vi "GenTest.vi"() -> ()   [LabVIEW 2017]
uses:
  DG822.lvlib
panel:
  out "Result":string
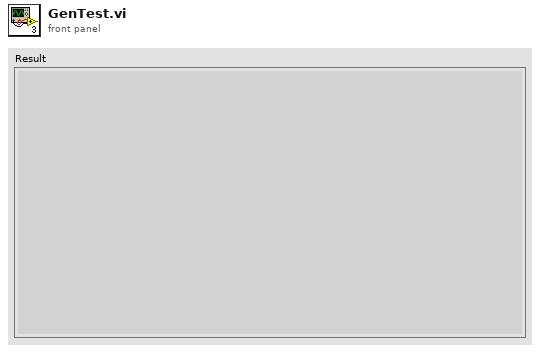
[diagram p1: front panel]
types:
  T1 = enum16{"SIN", "SQU", "RAMP", "PULSE", "NOISE", "HARM"}
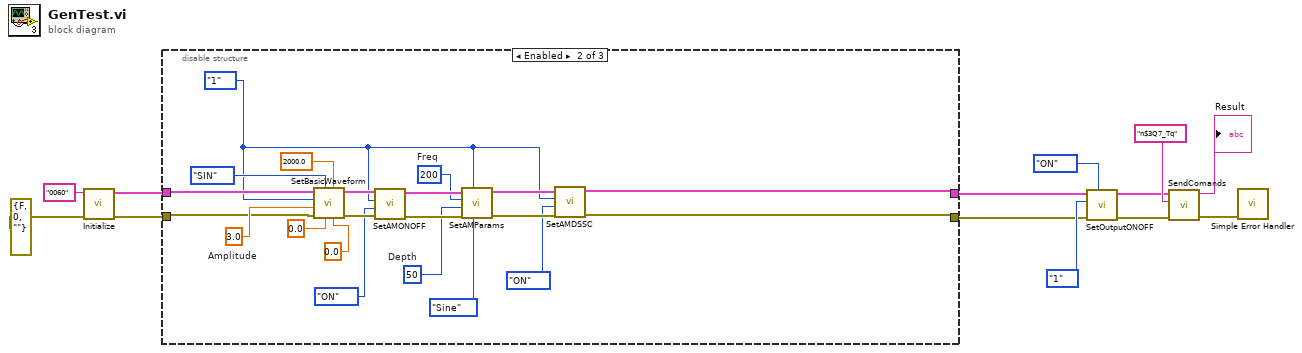
[diagram p0: block diagram]
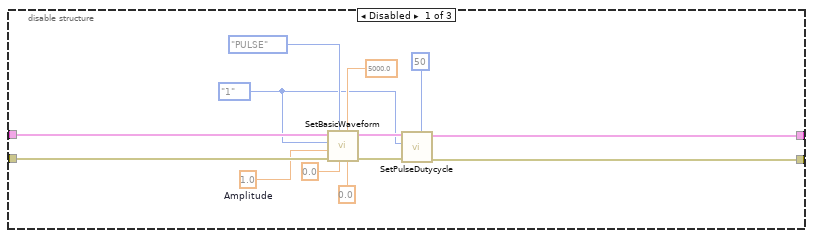
[diagram p2: hidden frame]
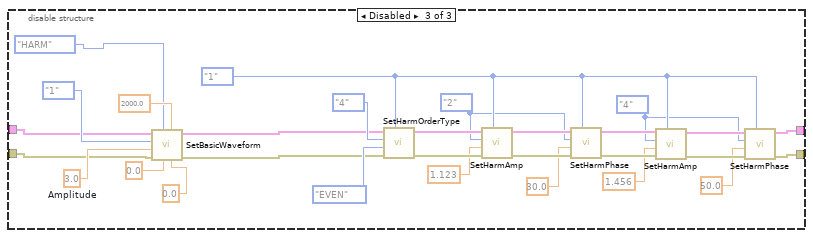
[diagram p3: hidden frame]
diagram:
  n1 = call "Initialize.vi"("error in (no error)"=errorcluster {"status"=FALSE, "code"=0, "source"=""}, "UserID"="0060") -> ("error out"=w7:errorcluster, "OutData"=w8:cluster{string, "userdata":string})  [unwired: 8 in]
  n2 = disable-structure shown="Enabled" {
    disable-tunnel: w8 -> [w26 w42 w53]
    disable-tunnel: w7 -> [w25 w41 w52]
    disable-tunnel: [w18 w34 w66] -> w2
    disable-tunnel: [w16 w33 w65] -> w1
    frame Disabled {
      w22 = 1.0  # Amplitude
      w15 = enum16{"1", "2"}."1" ("Source")
      n3 = call "SetBasicWaveform.vi"("Phase"=0.0, "Frequency"=5000.0, "Offset"=0.0, "Waveform"=enum16{"SIN", "SQU", "RAMP", "PULSE", "NOISE"}."PULSE", "error in"=w25, "Amplitude"=w22, "Source"=w15, "InputData"=w26) -> ("error out"=w17:errorcluster, "OutputData"=w19:cluster{"String":string, string})  [unwired: 2 in]
      n4 = call "SetPulseDutycycle.vi"("Dutycycle"=u8 50, "error in"=w17, "Source"=w15, "InputData"=w19) -> ("error out"=w16:errorcluster, "OutputData"=w18:cluster{"String":string, string})  [unwired: 6 in]
    }
    frame Enabled {
      w28 = u8 50  # Depth
      w30 = u32 200  # Freq
      w43 = 3.0  # Amplitude
      w32 = enum16{"1", "2"}."1" ("Source")
      n5 = call "SetBasicWaveform.vi"("Phase"=0.0, "Frequency"=2000.0, "Offset"=0.0, "Waveform"=T1."SIN", "error in"=w41, "Amplitude"=w43, "Source"=w32, "InputData"=w42) -> ("error out"=w39:errorcluster, "OutputData"=w40:cluster{"String":string, string})  [unwired: 2 in]
      n6 = call "SetAMONOFF.vi"("error in"=w39, "State"=enum16{"OFF", "ON"}."ON", "Source"=w32, "InputData"=w40) -> ("error out"=w37:errorcluster, "OutputData"=w38:cluster{"String":string, string})  [unwired: 6 in]
      n7 = call "SetAMParams.vi"("Func"=enum16{"Sine", "Square", "Trianle"}."Sine", "Source"=w32, "error in"=w37, "Depth"=w28, "Freq"=w30, "InputData"=w38) -> ("error out"=w35:errorcluster, "OutputData"=w36:cluster{"String":string, string})  [unwired: 4 in]
      n8 = call "SetAMDSSC.vi"("error in"=w35, "DSSC"=enum16{"OFF", "ON"}."ON", "Source"=w32, "InputData"=w36) -> ("error out"=w33:errorcluster, "OutputData"=w34:cluster{"String":string, string})  [unwired: 6 in]
    }
    frame Disabled {
      w55 = 3.0  # Amplitude
      w60 = enum16{"1", "2", "3", "4", "5"}."4" ("Harmonic")
      w63 = enum16{"1", "2", "3", "4", "5"}."2" ("Harmonic")
      w64 = enum16{"1", "2"}."1" ("Source")
      n9 = call "SetBasicWaveform.vi"("Phase"=0.0, "Frequency"=2000.0, "Offset"=0.0, "Waveform"=T1."HARM", "error in"=w52, "Amplitude"=w55, "Source"=enum16{"1", "2"}."1", "InputData"=w53) -> ("error out"=w48:errorcluster, "OutputData"=w49:cluster{"String":string, string})  [unwired: 2 in]
      n10 = call "SetHarmOrderType.vi"("Source"=w64, "error in"=w48, "Type"=enum16{"EVEN", "ODD", "BOTH"}."EVEN", "Order"=enum16{"1", "2", "3", "4", "5"}."4", "InputData"=w49) -> ("error out"=w75:errorcluster, "OutputData"=w76:cluster{"String":string, string})  [unwired: 5 in]
      n11 = call "SetHarmAmp.vi"("Source"=w64, "error in"=w75, "Amplitude"=1.123, "Harmonic"=w63, "InputData"=w76) -> ("error out"=w73:errorcluster, "OutputData"=w74:cluster{"String":string, string})  [unwired: 5 in]
      n12 = call "SetHarmPhase.vi"("Source"=w64, "error in"=w73, "Phase"=30.0, "Harmonic"=w63, "InputData"=w74) -> ("error out"=w67:errorcluster, "OutputData"=w68:cluster{"String":string, string})  [unwired: 5 in]
      n13 = call "SetHarmAmp.vi"("Source"=w64, "error in"=w67, "Amplitude"=1.456, "Harmonic"=w60, "InputData"=w68) -> ("error out"=w70:errorcluster, "OutputData"=w69:cluster{"String":string, string})  [unwired: 5 in]
      n14 = call "SetHarmPhase.vi"("Source"=w64, "error in"=w70, "Phase"=50.0, "Harmonic"=w60, "InputData"=w69) -> ("error out"=w65:errorcluster, "OutputData"=w66:cluster{"String":string, string})  [unwired: 5 in]
    }
  }
  n15 = call "SetOutputONOFF.vi"("State"=enum16{"OFF", "ON"}."ON", "error in"=w1, "Source"=enum16{"1", "2"}."1", "InputData"=w2) -> ("error out"=w5:errorcluster, "OutputData"=w6:cluster{"String":string, string})  [unwired: 6 in]
  n16 = call "SendComands.vi"("error in (no error)"=w5, "Password"="n$3Q7_Tq", "InputData"=w6) -> ("error out"=w9:errorcluster, "Result"=→"Result":string)  [unwired: 6 in, 1 out]
  n17 = call <vilib>:"Simple Error Handler.vi"("error in (no error)"=w9) -> ()  [unwired: 4 in, 5 out]
